vi "Set Mux.vi"(8 "error in (no error)":errorcluster, 10 "Mux Enabled Channels":bool[](array[boolean]), 11 "TCA9548A Mux in":refnum<class "TCA9548A I2C Multiplexer.lvclass">) -> (0 "error out":errorcluster, 3 "TCA9548A Mux out":refnum<class "TCA9548A I2C Multiplexer.lvclass">)   [LabVIEW 2020, in "CTI-Peripheral.lvlib" / "TCA9548A I2C Multiplexer.lvclass"]
uses:
  TCA9548A I2C Multiplexer.lvclass
  TCA9548A I2C Multiplexer.lvclass/TCA9548A I2C Multiplexer.ctl
  CTI/I2C Connection/I2C Connection.lvclass/I2C Connection.ctl
  CTI/Session/I2C Write Data.vi
  CTI/I2C Connection/I2C Connection.lvclass
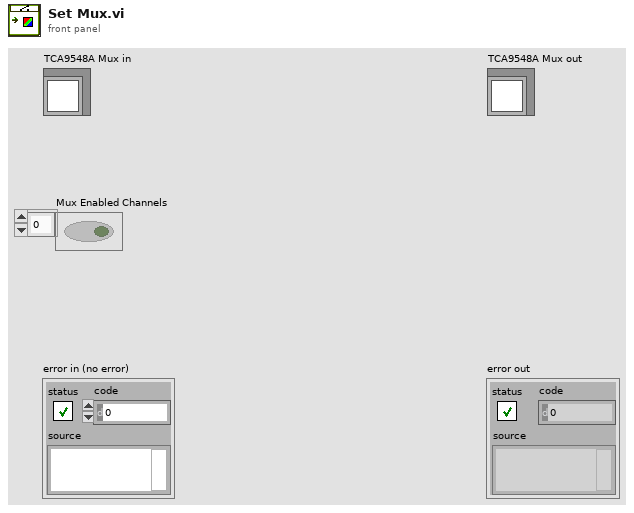
[diagram p1: front panel]
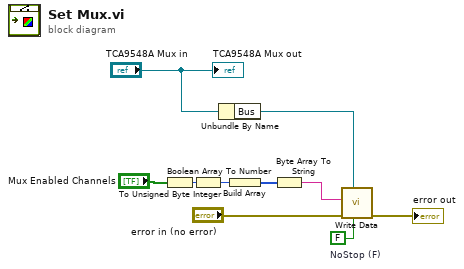
[diagram p0: block diagram]
diagram:
  w6 = FALSE  # NoStop (F)
  n1 = Boolean Array To Number(Boolean array="Mux Enabled Channels") -> (number=w3:u32)
  n2 = To Unsigned Byte Integer(number=w3) -> (unsigned 8bit integer=w1:u8)
  n3 = Unbundle By Name("TCA9548A Mux in") -> ("Bus"=w7:refnum<class "I2C Connection.lvclass">)
  n4 = Build Array(w1) -> (w10:u8[])
  n5 = Byte Array To String(unsigned byte array=w10) -> (string=w8:string)
  n6 = call "Write Data.vi"("NoStop (F)"=w6, "I2C Connection"=w7, "error in (no error)"="error in (no error)", "Data"=w8) -> ("error out"=→"error out":errorcluster)  [unwired: 7 in]
  "TCA9548A Mux out" <- "TCA9548A Mux in"
